vi "PH_Countdown-Counter.panel.vi"() -> ()   [LabVIEW 2014, in "PH_Countdown-Counter.lvlib"]
uses:
  PH_Countdown-Counter.lvlib
  PH_Basics/PH_Common/PH_Common.lvlib
  CS_Core/CSObj/CSObj.lvlib
  PH_Basics/PH_Class/PH_Class.lvlib
panel:
  in  "MainAmp only?":bool=TRUE
  in  "Exit":bool
  in  "Sound?":bool
  in  "Reminder 2":string="00:00:00"
  in  "Reminder 1":string="00:00:00"
  out "Remaining Time":string
  in  "Time between Shots":string="01:30:00"
  in  "Set Mode":bool caption="Mode"
  in  "Delete":bool
  out "error out":errorcluster
  in  "error in (no error)":errorcluster
  in  "object ref":refnum<vi>
  # "PCS"
  # "3.40"
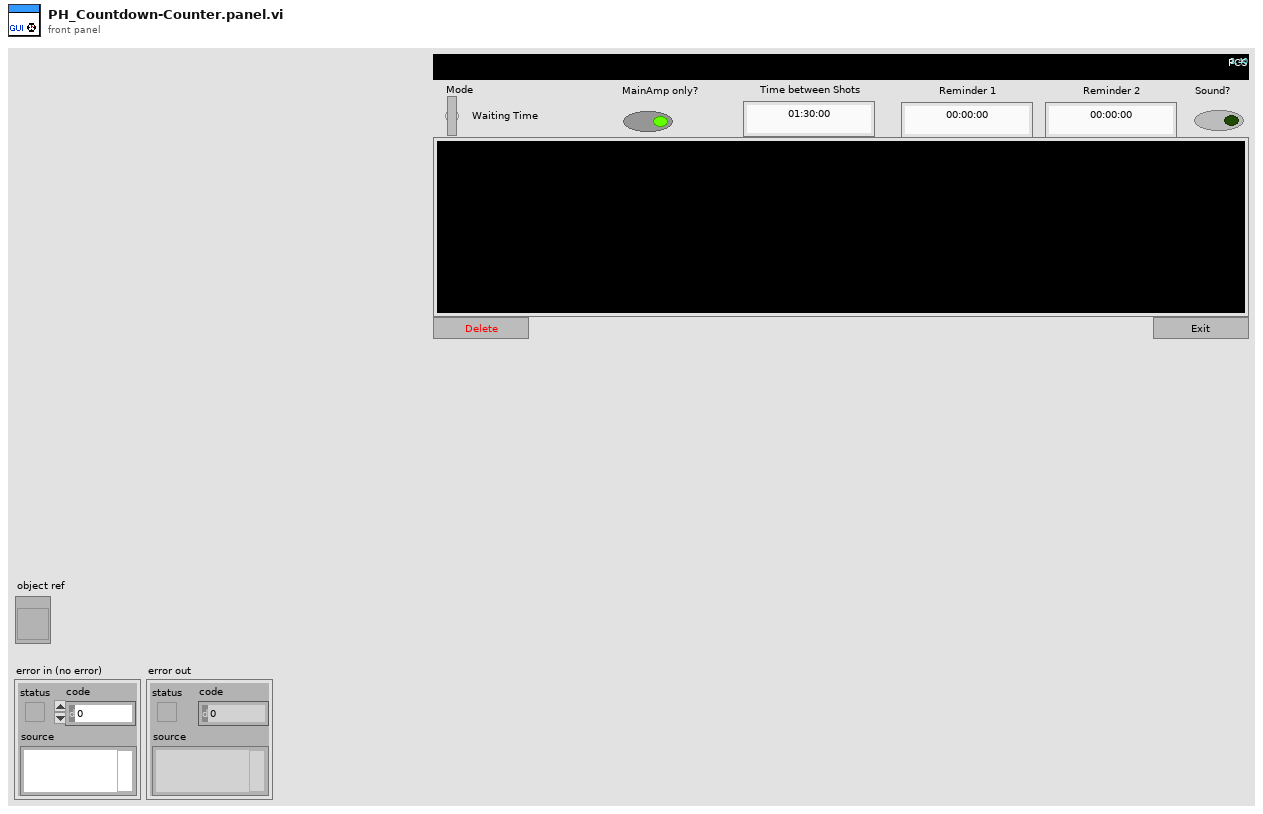
[diagram p1: front panel]
types:
  T1 = typedef "PH_Countdown-Counter.lvlib/PH_Countdown-Counter.i attribute.ctl" = cluster{"Machine Time":cluster{"Tag":string, "Wating Time [s]":dbl, "not linked?":bool}[], "Last Shot":cluster{"Tag":string, "Shot Time [s]":timestamp, "not linked?":bool}[], "Time since last Shot?":bool, "Calculation":cluster{"Time between Shots [s]":dbl, "Ref Remaining Time":refnum<vi>, "Service ID":i32, "over?":bool, "Ref Time between Shots":refnum<vi>, "Ref Set Mode":refnum<vi>}, "Sound?":bool, "Reminder":cluster{"# 1":cluster{"Pretime [s]":dbl, "Aktive?":bool, "Over?":bool}, "# 2":cluster{"Pretime [s]":dbl, "Aktive?":bool, "Over?":bool}}, "MainAmp only":cluster{"State":bool, "GUI Ref":refnum<vi>}}
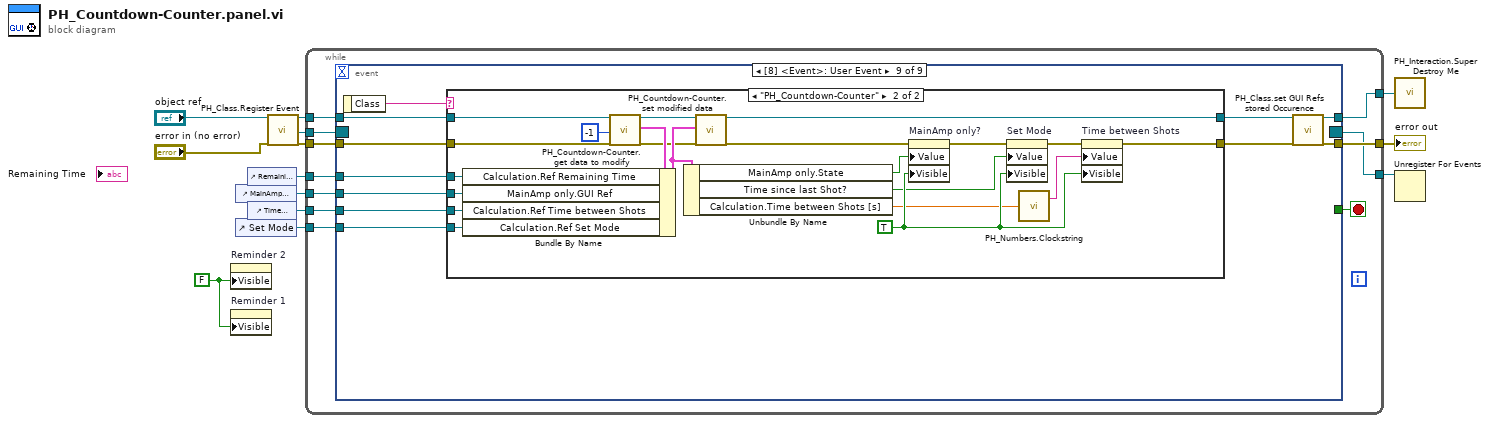
[diagram p0: block diagram]
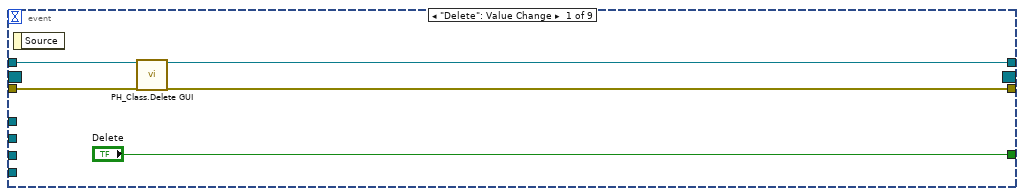
[diagram p2: hidden frame]
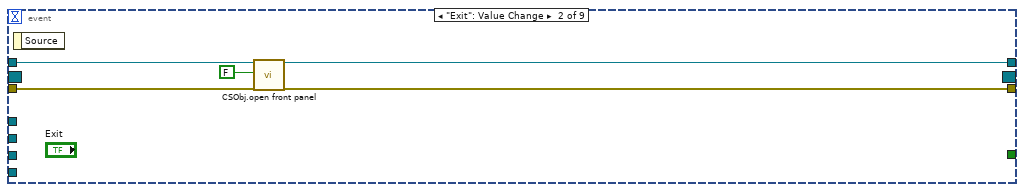
[diagram p3: hidden frame]
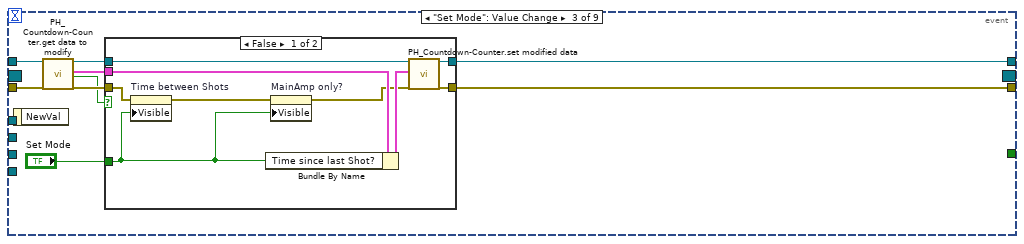
[diagram p4: hidden frame]
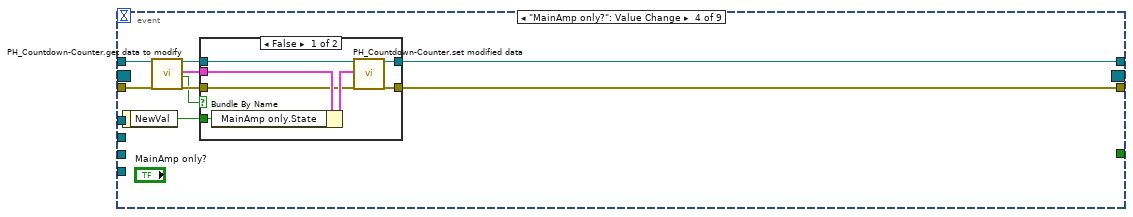
[diagram p6: hidden frame]
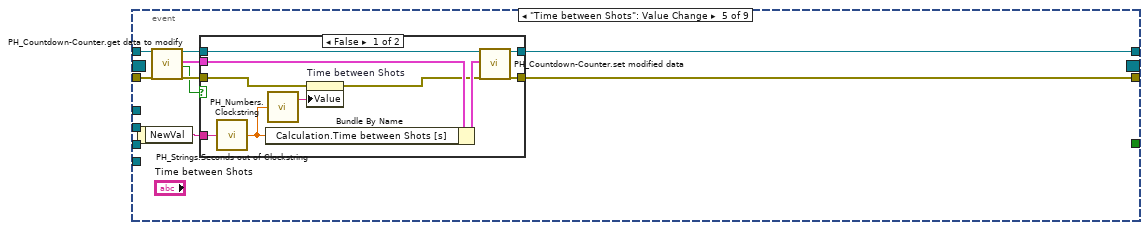
[diagram p8: hidden frame]
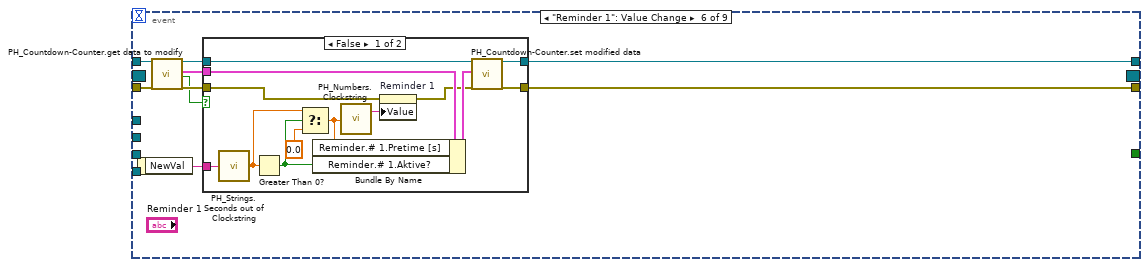
[diagram p10: hidden frame]
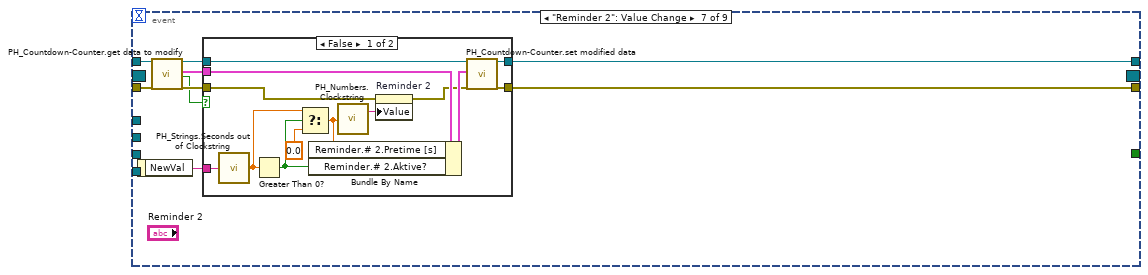
[diagram p12: hidden frame]
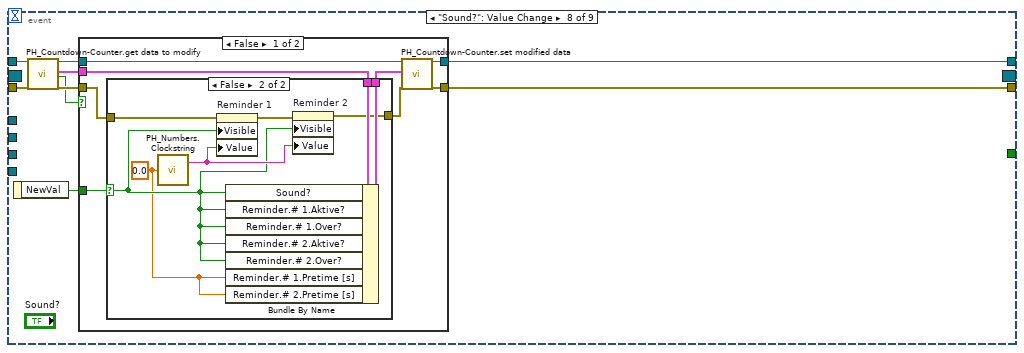
[diagram p14: hidden frame]
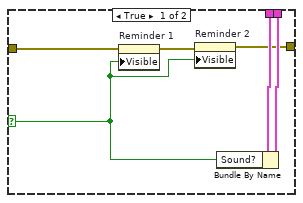
[diagram p15: hidden frame]
diagram:
  w11 = FALSE ("Visible")
  n1 = property on="Reminder 2" class="Str"("Visible"=w11) -> ()  [unwired: 2 in, 2 out]
  n2 = property on="Reminder 1" class="Str"("Visible"=w11) -> ()  [unwired: 2 in, 2 out]
  n3 = control-ref of="MainAmp only?"() -> (w3:refnum<vi>)
  n4 = control-ref of="Set Mode"() -> (w1:refnum<vi>)
  n5 = control-ref of="Remaining Time"() -> (w4:refnum<vi>)
  n6 = control-ref of="Time between Shots"() -> (w2:refnum<vi>)
  n7 = call "PH_Class.Register Event.vi"("i ref in"="object ref", "error in (no error)"="error in (no error)") -> ("i ref out"=w10:refnum<vi>, "Event Registration Refnum"=w8:refnum<event-registration>, "error out"=w9:errorcluster)  [unwired: 15 in]
  n8 = while {
    tunnel: w10 -> [w21]
    tunnel: [w20] -> w13
    tunnel: [w23] -> w12
    tunnel: w9 -> [w22]
    tunnel: w8 -> [w19]
    tunnel: [w18] -> w7
    tunnel: w4 -> [w17]
    tunnel: w3 -> [w16]
    tunnel: w2 -> [w15]
    tunnel: w1 -> [w14]
    stop <- w24 stop-if-true
    n9 = event shown="[8] <Event>: User Event" {
      selector: w19 -> [_ _ _ _ _ _ _ _ _]
      dyn-events: [_ _ _ _ _ _ _ _ _] -> w18
      timeout: _ -> [_ _ _ _ _ _ _ _ _]
      tunnel: ["Delete" _ _ _ _ _ _ _ _] -> w24
      tunnel: w21 -> [w28 w33 w40 w60 w78 w99 w123 w147 w185]
      tunnel: [w25 w30 w37 w57 w75 w96 w120 w144 w182] -> w23
      tunnel: w22 -> [w27 w31 w41 w61 w79 w100 w124 w148 w181]
      tunnel: [w26 w32 w36 w56 w74 w95 w119 w143 w183] -> w20
      tunnel: w17 -> [_ _ _ _ _ _ _ _ w179]
      tunnel: w16 -> [_ _ _ _ _ _ _ _ w178]
      tunnel: w15 -> [_ _ _ _ _ _ _ _ w177]
      tunnel: w14 -> [_ _ _ _ _ _ _ _ w176]
      event "Delete": Value Change {
        n10 = event-data() -> ()  [unwired: 1 in, 1 out]
        n11 = call "PH_Class.Delete GUI.vi"("VI in"=w28, "error in (no error)"=w27) -> ("VI out"=w26:refnum<vi>, "error out"=w25:errorcluster)  [unwired: 16 in]
      }
      event "Exit": Value Change {
        n12 = event-data() -> ()  [unwired: 1 in, 1 out]
        n13 = call "CSObj.open front panel.vi"("i ref in"=w33, "frontPanelOpen"=FALSE ("front panel open"), "error in (no error)"=w31) -> ("i ref out"=w32:refnum<vi>, "error out"=w30:errorcluster)  [unwired: 15 in]
      }
      event "Set Mode": Value Change {
        n14 = event-data() -> ()  [unwired: 1 in, 1 out]
        n15 = call "PH_Countdown-Counter.get data to modify.vi"("i ref in"=w40, "error in (no error)"=w41) -> ("i ref out"=w42:refnum<vi>, "i attribute"=w39:T1, "timed out"=w38:bool, "error out"=w43:errorcluster)  [unwired: 14 in]
        n16 = case shown="False" w38 {
          tunnel: w43 -> [w47 w53]
          tunnel: w42 -> [w52 w54]
          tunnel: [w51 w53] -> w37
          tunnel: [w50 w54] -> w36
          tunnel: w39 -> [w49 _]
          tunnel: "Set Mode" -> [w44 _]
          frame False {
            n17 = property on="Time between Shots" class="Str"(error in=w47, "Visible"=w44) -> (error out=w46:errorcluster)  [unwired: 1 in, 1 out]
            n18 = Bundle By Name(cluster=w49, "Time since last Shot?"=w44) -> (w48:T1)
            n19 = property on="MainAmp only?" class="Bool (strict)"(error in=w46, "Visible"=w44) -> (error out=w45:errorcluster)  [unwired: 1 in, 1 out]
            n20 = call "PH_Countdown-Counter.set modified data.vi"("i ref in"=w52, "i attribute"=w48, "error in (no error)"=w45) -> ("i ref out"=w50:refnum<vi>, "error out"=w51:errorcluster)  [unwired: 15 in]
          }
          frame True {
          }
        }
      }
      event "MainAmp only?": Value Change {
        n21 = event-data() -> ("NewVal"=w55:bool)  [unwired: 1 in]
        n22 = call "PH_Countdown-Counter.get data to modify.vi"("i ref in"=w60, "error in (no error)"=w61) -> ("i ref out"=w62:refnum<vi>, "i attribute"=w59:T1, "timed out"=w58:bool, "error out"=w63:errorcluster)  [unwired: 14 in]
        n23 = case shown="False" w58 {
          tunnel: w63 -> [w64 w71]
          tunnel: w62 -> [w70 w72]
          tunnel: [w69 w71] -> w57
          tunnel: [w68 w72] -> w56
          tunnel: w59 -> [w67 _]
          tunnel: w55 -> [w65 _]
          frame False {
            n24 = Bundle By Name(cluster=w67, "MainAmp only.State"=w65) -> (w66:T1)
            n25 = call "PH_Countdown-Counter.set modified data.vi"("i ref in"=w70, "i attribute"=w66, "error in (no error)"=w64) -> ("i ref out"=w68:refnum<vi>, "error out"=w69:errorcluster)  [unwired: 15 in]
          }
          frame True {
          }
        }
      }
      event "Time between Shots": Value Change {
        n26 = event-data() -> ("NewVal"=w73:string)  [unwired: 1 in]
        n27 = call "PH_Countdown-Counter.get data to modify.vi"("i ref in"=w78, "error in (no error)"=w79) -> ("i ref out"=w80:refnum<vi>, "i attribute"=w77:T1, "timed out"=w76:bool, "error out"=w81:errorcluster)  [unwired: 14 in]
        n28 = case shown="False" w76 {
          tunnel: w81 -> [w85 w92]
          tunnel: w80 -> [w91 w93]
          tunnel: [w90 w92] -> w75
          tunnel: [w89 w93] -> w74
          tunnel: w77 -> [w88 _]
          tunnel: w73 -> [w86 _]
          frame False {
            n29 = call "PH_Strings.Seconds out of Clockstring.vi"("Clock String"=w86) -> ("Time [s]"=w83:dbl)
            n30 = Bundle By Name(cluster=w88, "Calculation.Time between Shots [s]"=w83) -> (w87:T1)
            n31 = call "PH_Numbers.Clockstring.vi"("Time [s]"=w83) -> ("Clock String"=w82:string)  [unwired: 1 out]
            n32 = property on="Time between Shots" class="Str"(error in=w85, "Value"=w82) -> (error out=w84:errorcluster)  [unwired: 1 in, 1 out]
            n33 = call "PH_Countdown-Counter.set modified data.vi"("i ref in"=w91, "i attribute"=w87, "error in (no error)"=w84) -> ("i ref out"=w89:refnum<vi>, "error out"=w90:errorcluster)  [unwired: 15 in]
          }
          frame True {
          }
        }
      }
      event "Reminder 1": Value Change {
        n34 = event-data() -> ("NewVal"=w94:string)  [unwired: 1 in]
        n35 = call "PH_Countdown-Counter.get data to modify.vi"("i ref in"=w99, "error in (no error)"=w100) -> ("i ref out"=w101:refnum<vi>, "i attribute"=w98:T1, "timed out"=w97:bool, "error out"=w102:errorcluster)  [unwired: 14 in]
        n36 = case shown="False" w97 {
          tunnel: w102 -> [w109 w116]
          tunnel: w101 -> [w115 w117]
          tunnel: [w114 w116] -> w96
          tunnel: [w113 w117] -> w95
          tunnel: w98 -> [w112 _]
          tunnel: w94 -> [w110 _]
          frame False {
            n37 = call "PH_Strings.Seconds out of Clockstring.vi"("Clock String"=w110) -> ("Time [s]"=w105:dbl)
            n38 = Greater Than 0?(x=w105) -> (x > 0?=w106:bool)
            n39 = Select(t=w105, s=w106, f=0.0) -> (s? t:f=w104:dbl)
            n40 = Bundle By Name(cluster=w112, "Reminder.# 1.Pretime [s]"=w104, "Reminder.# 1.Aktive?"=w106) -> (w111:T1)
            n41 = call "PH_Numbers.Clockstring.vi"("Time [s]"=w104) -> ("Clock String"=w107:string)  [unwired: 1 out]
            n42 = property on="Reminder 1" class="Str"(error in=w109, "Value"=w107) -> (error out=w108:errorcluster)  [unwired: 1 in, 1 out]
            n43 = call "PH_Countdown-Counter.set modified data.vi"("i ref in"=w115, "i attribute"=w111, "error in (no error)"=w108) -> ("i ref out"=w113:refnum<vi>, "error out"=w114:errorcluster)  [unwired: 15 in]
          }
          frame True {
          }
        }
      }
      event "Reminder 2": Value Change {
        n44 = event-data() -> ("NewVal"=w118:string)  [unwired: 1 in]
        n45 = call "PH_Countdown-Counter.get data to modify.vi"("i ref in"=w123, "error in (no error)"=w124) -> ("i ref out"=w125:refnum<vi>, "i attribute"=w122:T1, "timed out"=w121:bool, "error out"=w126:errorcluster)  [unwired: 14 in]
        n46 = case shown="False" w121 {
          tunnel: w126 -> [w129 w140]
          tunnel: w125 -> [w139 w141]
          tunnel: [w138 w140] -> w120
          tunnel: [w137 w141] -> w119
          tunnel: w122 -> [w136 _]
          tunnel: w118 -> [w134 _]
          frame False {
            n47 = call "PH_Strings.Seconds out of Clockstring.vi"("Clock String"=w134) -> ("Time [s]"=w132:dbl)
            n48 = Greater Than 0?(x=w132) -> (x > 0?=w133:bool)
            n49 = Select(t=w132, s=w133, f=0.0) -> (s? t:f=w131:dbl)
            n50 = Bundle By Name(cluster=w136, "Reminder.# 2.Pretime [s]"=w131, "Reminder.# 2.Aktive?"=w133) -> (w135:T1)
            n51 = call "PH_Numbers.Clockstring.vi"("Time [s]"=w131) -> ("Clock String"=w127:string)  [unwired: 1 out]
            n52 = property on="Reminder 2" class="Str"(error in=w129, "Value"=w127) -> (error out=w128:errorcluster)  [unwired: 1 in, 1 out]
            n53 = call "PH_Countdown-Counter.set modified data.vi"("i ref in"=w139, "i attribute"=w135, "error in (no error)"=w128) -> ("i ref out"=w137:refnum<vi>, "error out"=w138:errorcluster)  [unwired: 15 in]
          }
          frame True {
          }
        }
      }
      event "Sound?": Value Change {
        n54 = event-data() -> ("NewVal"=w142:bool)  [unwired: 1 in]
        n55 = call "PH_Countdown-Counter.get data to modify.vi"("i ref in"=w147, "error in (no error)"=w148) -> ("i ref out"=w149:refnum<vi>, "i attribute"=w146:T1, "timed out"=w145:bool, "error out"=w150:errorcluster)  [unwired: 14 in]
        n56 = case shown="False" w145 {
          tunnel: w150 -> [w153 w173]
          tunnel: w149 -> [w158 w174]
          tunnel: [w157 w173] -> w144
          tunnel: [w156 w174] -> w143
          tunnel: w146 -> [w155 _]
          tunnel: w142 -> [w151 _]
          frame False {
            n57 = case shown="False" w151 {
              selector: w151 -> [w159 w166]
              tunnel: w155 -> [w164 w172]
              tunnel: [w163 w171] -> w154
              tunnel: w153 -> [w161 w169]
              tunnel: [w160 w168] -> w152
              frame True {
                n58 = property on="Reminder 1" class="Str"(error in=w161, "Visible"=w159) -> (error out=w162:errorcluster)  [unwired: 1 in, 1 out]
                n59 = property on="Reminder 2" class="Str"(error in=w162, "Visible"=w159) -> (error out=w160:errorcluster)  [unwired: 1 in, 1 out]
                n60 = Bundle By Name(cluster=w164, "Sound?"=w159) -> (w163:T1)
              }
              frame False {
                w165 = 0.0 ("Time [s]")
                n61 = call "PH_Numbers.Clockstring.vi"("Time [s]"=w165) -> ("Clock String"=w167:string)  [unwired: 1 out]
                n62 = property on="Reminder 1" class="Str"(error in=w169, "Visible"=w166, "Value"=w167) -> (error out=w170:errorcluster)  [unwired: 1 in, 1 out]
                n63 = Bundle By Name(cluster=w172, "Sound?"=w166, "Reminder.# 1.Aktive?"=w166, "Reminder.# 1.Over?"=w166, "Reminder.# 2.Aktive?"=w166, "Reminder.# 2.Over?"=w166, "Reminder.# 1.Pretime [s]"=w165, "Reminder.# 2.Pretime [s]"=w165) -> (w171:T1)
                n64 = property on="Reminder 2" class="Str"(error in=w170, "Visible"=w166, "Value"=w167) -> (error out=w168:errorcluster)  [unwired: 1 in, 1 out]
              }
            }
            n65 = call "PH_Countdown-Counter.set modified data.vi"("i ref in"=w158, "i attribute"=w154, "error in (no error)"=w152) -> ("i ref out"=w156:refnum<vi>, "error out"=w157:errorcluster)  [unwired: 15 in]
          }
          frame True {
          }
        }
      }
      event User Event {
        n66 = event-data() -> ("Class"=w175:string)  [unwired: 1 in]
        n67 = case shown="\"PH_Countdown-Counter\"" w175 {
          tunnel: w185 -> [w187 w195]
          tunnel: [w187 w194] -> w184
          tunnel: w181 -> [w186 w193]
          tunnel: [w186 w192] -> w180
          tunnel: w179 -> [_ w191]
          tunnel: w178 -> [_ w190]
          tunnel: w177 -> [_ w189]
          tunnel: w176 -> [_ w188]
          frame Default {
          }
          frame "PH_Countdown-Counter" {
            w208 = TRUE ("Visible")
            n68 = call "PH_Countdown-Counter.get data to modify.vi"("i ref in"=w195, "ms timeout (10000)"=-1, "error in (no error)"=w193) -> ("i ref out"=w198:refnum<vi>, "i attribute"=w199:T1, "error out"=w196:errorcluster)  [unwired: 13 in, 1 out]
            n69 = Bundle By Name(cluster=w199, "Calculation.Ref Remaining Time"=w191, "MainAmp only.GUI Ref"=w190, "Calculation.Ref Time between Shots"=w189, "Calculation.Ref Set Mode"=w188) -> (w200:T1)
            n70 = Unbundle By Name(w200) -> ("MainAmp only.State"=w201:bool, "Time since last Shot?"=w204:bool, "Calculation.Time between Shots [s]"=w205:dbl)
            n71 = call "PH_Countdown-Counter.set modified data.vi"("i ref in"=w198, "i attribute"=w200, "error in (no error)"=w196) -> ("i ref out"=w194:refnum<vi>, "error out"=w202:errorcluster)  [unwired: 15 in]
            n72 = property on="MainAmp only?" class="Bool (strict)"(error in=w202, "Value"=w201, "Visible"=w208) -> (error out=w203:errorcluster)  [unwired: 1 in, 1 out]
            n73 = property on="Set Mode" class="Bool (strict)"(error in=w203, "Value"=w204, "Visible"=w208) -> (error out=w206:errorcluster)  [unwired: 1 in, 1 out]
            n74 = call "PH_Numbers.Clockstring.vi"("Time [s]"=w205) -> ("Clock String"=w207:string)  [unwired: 1 out]
            n75 = property on="Time between Shots" class="Str"(error in=w206, "Value"=w207, "Visible"=w208) -> (error out=w192:errorcluster)  [unwired: 1 in, 1 out]
          }
        }
        n76 = call "PH_Class.set GUI Refs stored Occurence.vi"("i ref in"=w184, "error in (no error)"=w180) -> ("i ref out"=w183:refnum<vi>, "error out"=w182:errorcluster)  [unwired: 16 in]
      }
    }
  }
  "error out" <- w12
  n77 = call "PH_Interaction.Super Destroy Me.vi"("i ref out"=w13) -> ()
  n78 = Unregister For Events(event registration refnum=w7) -> ()  [unwired: 1 in, 1 out]
